vi "Handle Error.vi"(8 "error in (no error)":errorcluster, 11 "HIJ File Viewer Demo App in":refnum<class "HIJ File Viewer Demo App.lvclass">) -> (0 "error out":errorcluster, 2 "stop actor?":bool=TRUE, 3 "HIJ File Viewer Demo App out":refnum<class "HIJ File Viewer Demo App.lvclass">)   [LabVIEW 2014, in "HIJ File Viewer Demo App.lvlib" / "HIJ File Viewer Demo App.lvclass"]
doc: "(<B>Filename</B>: Actor Framework.lvlib:Actor.lvclass:Handle Error.vi)\n\nDefines how the actor handles an error that occurred while processing a message. By default, this method does nothing except stop the actor."
uses:
  HIJ File Viewer Demo App.lvclass
  Applications/Launch HIJ FileViewer/HIJ Vision File Viewer App/HIJ Vision File Viewer App.lvclass
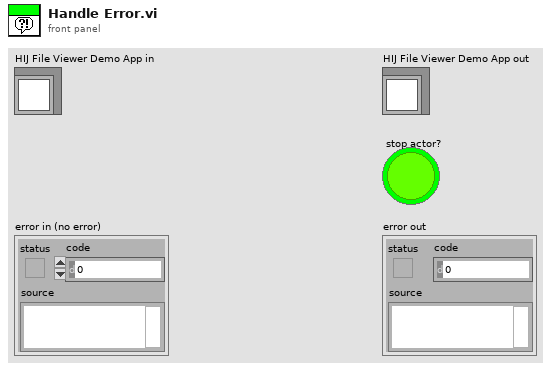
[diagram p1: front panel]
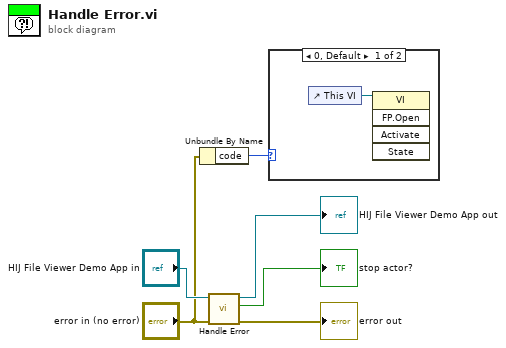
[diagram p0: block diagram]
diagram:
  n1 = Unbundle By Name("error in (no error)") -> ("code"=w1:i32)
  n2 = call-parent "Handle Error.vi"("error in (no error)"="error in (no error)", "Actor in"="HIJ File Viewer Demo App in") -> ("error out"=→"error out":errorcluster, "stop actor?"=→"stop actor?":bool, "Actor out"=→"HIJ File Viewer Demo App out":refnum<class "HIJ File Viewer Demo App.lvclass">)  [unwired: 7 in]
  n3 = case shown="0, Default" w1 {
    frame 0, Default {
      n4 = control-ref of="This VI"() -> (w7:refnum<vi>)
      n5 = invoke class="VI" method="FP.Open"(reference=w7) -> ()  [unwired: 4 in, 5 out]
    }
    frame 43 {
    }
  }
